vi "Get Theme Colors.vi"(8 "error in (no error)":errorcluster, 11 "Filled Text Fields in":refnum<class "Filled Text Fields.lvclass">) -> (0 "error out":errorcluster, 2 "Properties:Colors":T1={"Main"={"Primary"=15224622, "Primary Variant"=16744512, "Secondary"=9342606, "Secondary Varient"=2039583}, "Container"={"BG"=16119285, "Hover"=15527148, "Focused"=14474460}, "Text"={"Default"=5855577, "Error"=11534368}}, 3 "Filled Text Fields out":refnum<class "Filled Text Fields.lvclass">)   [LabVIEW 2017, in "Filled Text Fields.lvlib" / "Filled Text Fields.lvclass"]
uses:
  Filled Text Fields.lvclass
  Theme/Theme.Colors/Colors.ctl
  Filled Text Fields.lvclass/Filled Text Fields.ctl
  Theme/Theme/getColors.vi
  Theme/Theme/Theme.lvclass
  Theme/Theme.Colors/Theme.Colors.lvclass
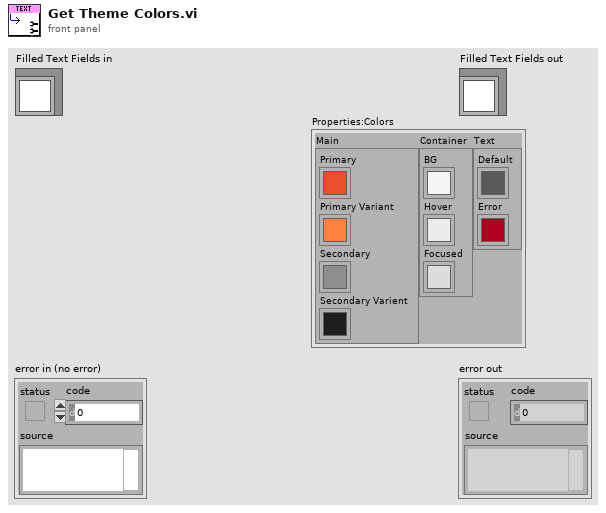
[diagram p1: front panel]
types:
  T1 = typedef "Theme.lvlib/Theme.Colors.lvclass/Colors.ctl" = cluster{"Main":cluster{"Primary":u32, "Primary Variant":u32, "Secondary":u32, "Secondary Varient":u32}, "Container":cluster{"BG":u32, "Hover":u32, "Focused":u32}, "Text":cluster{"Default":u32, "Error":u32}}
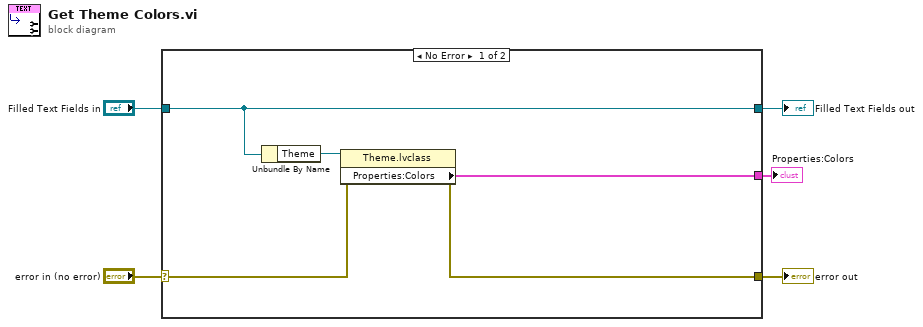
[diagram p0: block diagram]
diagram:
  n1 = case shown="No Error" "error in (no error)" {
    selector: "error in (no error)" -> [w7 w12]
    tunnel: [w6 w12] -> w4
    tunnel: [w10 w11] -> w2
    tunnel: "Filled Text Fields in" -> [w10 w11]
    tunnel: [w8 _] -> w1
    frame No Error {
      n2 = Unbundle By Name(w10) -> ("Theme"=w9:refnum<class "Theme.lvclass">)
      n3 = property class="Theme.lvclass"(reference=w9, error in=w7) -> (error out=w6:errorcluster, "Properties:Colors"=w8:T1)  [unwired: 1 out]
    }
    frame Error {
    }
  }
  "error out" <- w4
  "Filled Text Fields out" <- w2
  "Properties:Colors" <- w1
